vi "CsTool-QueryAcquisitionParametersFill.vi"(11 "Handle Cluster":T2) -> (0 "Error Code":i32, 1 "Trigger Delay":dbl, 2 "Trigger Holdoff":dbl, 3 "Trigger Timeout":dbl, 4 "Depth":dbl, 5 "Segment Count":u32, 6 "Output Handle Cluster":T1, 7 "Segment Size":dbl, 8 "Mode":string, 9 "Clock Mode":enum16{"Internal", "External", "Reference"}(ring), 10 "Sample Rate":dbl)   [LabVIEW 2022 SP3]
doc: "This VI returns the acquisition configuration settings that have been set in the driver for the system identified by Handle Cluster, which is obtained by using CsTool-GetSystem.vi. If the call cannot be completed, an appropriate error code is returned. A descriptive error string may be obtained by calling CsTool-ErrorHandler.vi.\n\nThe returned acquisition configuration settings are: Sample Rate, Clock Mode, Mode, Segment Count, Depth, Segment Size, Trigger Timeout, Trigger Holdoff and Trigger Delay. An Output Handle Cluster is also returned. The returned values are those that were successfully set on the CompuScope hardware by the last call to CsTool-Commit.vi. The returned values are not valid until CsTool-Commit.vi has been called at least once. \n\n\nReturn Value Descriptions:\n\nSample Rate\nThis double variable value is the rate at which the CompuScope system will sample the input waveform. It is specified in Samples per second. \n\nClock Mode\nThis integer value is returned as 0 if the system is using Internal clocking, 1 if it is using External clocking, and 2 if it is using the 10 MHz Reference clocking.\n\nMode\nThis string value indicates the current operating mode for the CompuScope system. Possible values are:\n single\n dual\n quad\n octal\n\nNote that for digital input CompuScope cards, like the CS3200 and CS3200C, \"single\" is equivalent to 8-bit mode, \"dual\" is equivalent to 16-bit mode and \"quad\" is equivalent to 32-bit mode.\n\nSegment Count \nThis integer value indicates how many segments (or records) will be captured in a Multiple Record acquisition. For Single Record acquisitions, the variable is always returned as 1. \n\nDepth \nThis double variable value indicates the number of post-trigger samples that the CompuScope system is set to acquire. \n\nSegment Size\nThis double variable indicates the total amount of memory allocated to the acquisition. The maximum possible amount of pre-trigger data that can be acquired, therefore, is (Segment Size - Depth). \n\nTrigger Timeout\nThis double variable value indicates the amount of time that the CompuScope system will wait before forcing a trigger. The value is in microseconds. \n\nTrigger Delay\nThis double variable value indicates the number of Samples between the time that the trigger event actually occurs and the time that the trigger event will be logged in the data record. Setting a non-zero trigger delay is useful for signals where the region of interest in the signal occurs long after the trigger event. Trigger Delay is not supported on all CompuScope models.\n\nTrigger Holdoff\nThis double variable value indicates the amount of time in Samples during which the CompuScope hardware will ignore trigger events after beginning an acquisition. Trigger Holdoff is useful in order to ensure the accumulation of specified number of pre-trigger points by ignoring trigger events until the specified number has been acquired. \n\nOutput Handle Cluster\nThe Output Handle Cluster is provided in order to correctly account for the presence of optional CompuScope firmware, which may cause changes to the CompuScope data format. The Handle Cluster provided by CsTool-GetSystem only applies for the CompuScope system using standard on-board firmware. Optional firmware, however, may change the sample data format, for example, from 16-bit samples to 32-bit samples. Because of this, CsTool-QueryAcquistionParameters provides the Output Handle Cluster, which accounts for any data format changes due to optional firmware. The Output Handle Cluster contains the Sample Size, Sample Resolution and Sample Offset updated to account for optional firmware."
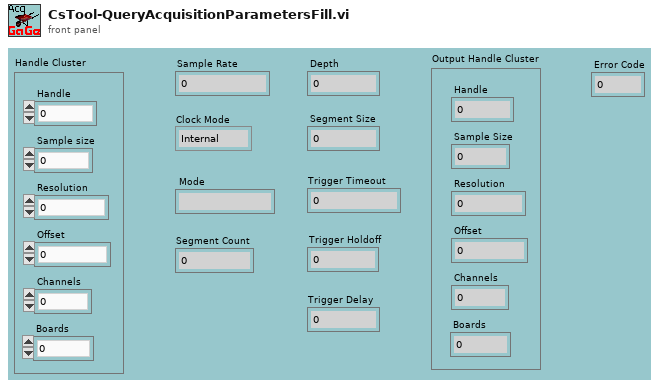
[diagram p1: front panel]
types:
  T1 = cluster{"Handle":u32, "Sample Size":u32, "Resolution":i32, "Offset":i32, "Channels":u32, "Boards":u32}
  T2 = cluster{"Handle":u32, "Sample size":u32, "Resolution":i32, "Offset":i32, "Channels":u32, "Boards":u32}
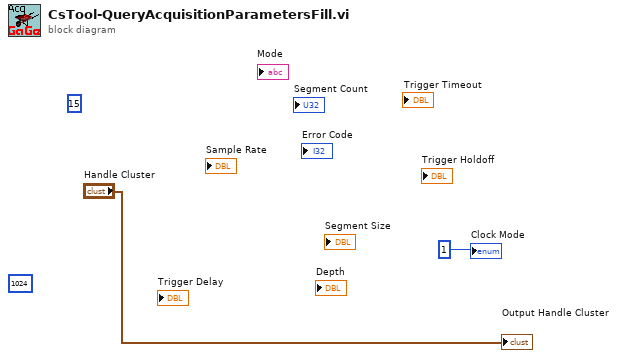
[diagram p0: block diagram]
diagram:
  (unwired) 1024
  (unwired) 15
  "Output Handle Cluster" <- "Handle Cluster"
  "Clock Mode" <- 1
